vi "ICmainProgram.vi"() -> ()   [LabVIEW 2018]
uses:
  NetworkStream/NetworkStreamReceiverState.ctl
  NetworkStream/NetworkStreamData.ctl
  <vilib>/vision/Image Controls.llb/IMAQ Image.ctl
  NetworkStream/NetworkStreamStateMachineVariable.ctl
  <vilib>/dex/Stream Element Allocation Mode.ctl
  Shared program Control/MasterStatus.ctl
  StateMachine.ctl
  General Libraries/Photon Filtering.lvlib
  NetworkStream/NetworkStream.lvlib
  Tektronik3102/TektronikNetwork.lvlib
  Shared program Control/MySharedVariables.lvlib
panel:
  out "Network Stream State Indicator":T1
  out "output cluster":T2
  out "Session Hash":u64
  in  "Tab Control":enum32{"Camera", "Trigger", "configuration"}(tab)
  in  "exposure (us)":i32(slide) caption="exposure" scale=50.0..30000000.0
  in  "gain":i32(slide) scale=32.0..2047.0
  in  "sofware trigger":bool
  in  "live":bool
  in  "Save":bool
  in  "Trigger ON":bool
  out "Sequence Number":u64
  in  "Save Folder Path":path=path "D:/Data/Mai/test target"
  in  "VCD Properties":bool
  in  "Stop Button":bool
  out "error out":errorcluster
  in  "?":enum32{"IC control", "Data analysis", "graphs"}(tab)
  in  "ICImagingControl":refnum<k7>(container)
  out "Image":T3(plugin-control)
  in  "flush queue":bool
  in  "Flush Pile":bool
  in  "Mask ON":bool
  out "filtered \nFFT":dbl[][](graph)
  out "FFT":dbl[][](graph)
  in  "save image":bool
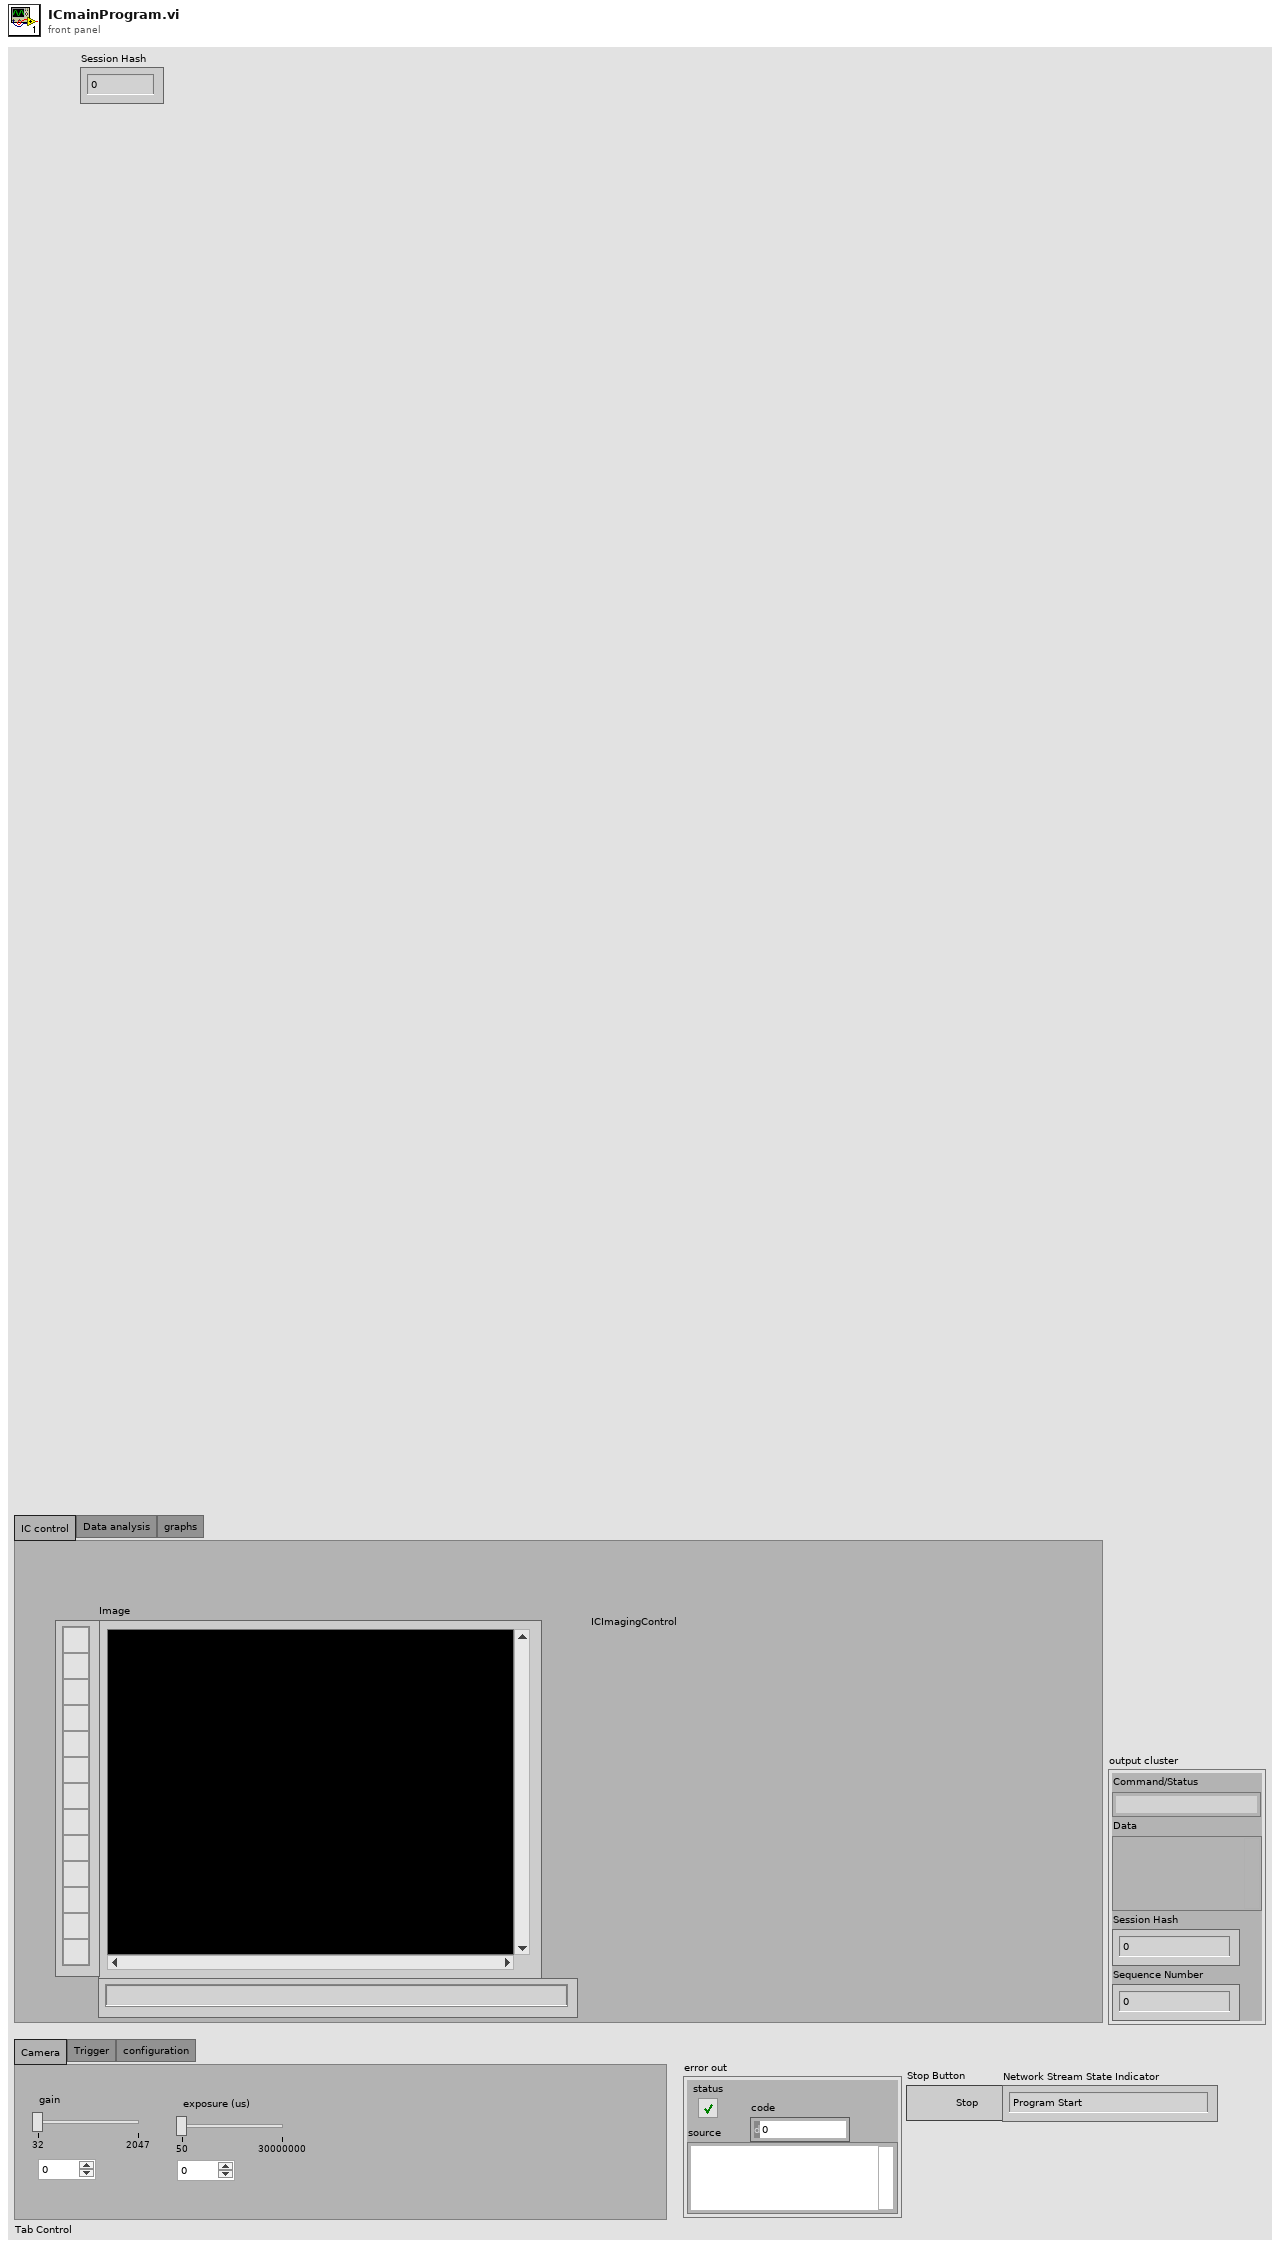
[diagram p1: front panel]
types:
  T1 = typedef "NetworkStream.lvlib/NetworkStreamReceiverState.ctl" = enum16{"Program Start", "Waiting for connection", "Connected", "Connection lost", "Exit", "Unhandled Exception"}
  T2 = typedef "NetworkStream.lvlib/NetworkStreamData.ctl" = cluster{"Command/Status":string, "Data":variant, "Session Hash":u64, "Sequence Number":u64}
  T3 = typedef "IMAQ Image.ctl" = refnum<image>
  T4 = typedef "NetworkStream.lvlib/NetworkStreamStateMachineVariable.ctl" = cluster{"Network Stream Reader Endpoint":refnum<k21>, "Last Received Sequence Number":u64}
  T5 = typedef "MySharedVariables.lvlib/MasterStatus.ctl" = cluster{"Camera done":bool, "Tektronik done":bool, "Motors done":bool, "Gage done":bool}[]
  T6 = cluster{"Image Out":T3, "Start time":dbl, "Stop time":dbl, "Index":i32}
  T7 = typedef "Stream Element Allocation Mode.ctl" = u32
  T8 = enum16{"Brightness", "Color Enable", "Contrast", "Exposure", "Focus", "Gain", "Gamma", "Hue", "Iris", "Pan", "Roll", "Saturation", "Sharpness", "Tilt", "Whitebalance", "Zoom", "Whitebalance Blue", "Whitebalance Red"}
  T9 = cluster{"Rows Per Strip":i32, "Photometric":i32, "Compression Type":i32}
  T10 = typedef "StateMachine.ctl" = enum16{"free running", "sequence recording", "run statistics"}
  T11 = cluster{"Image Out":T3, "SampleStartTime":dbl, "SampleEndTime":dbl, "Sequence Number":u64}
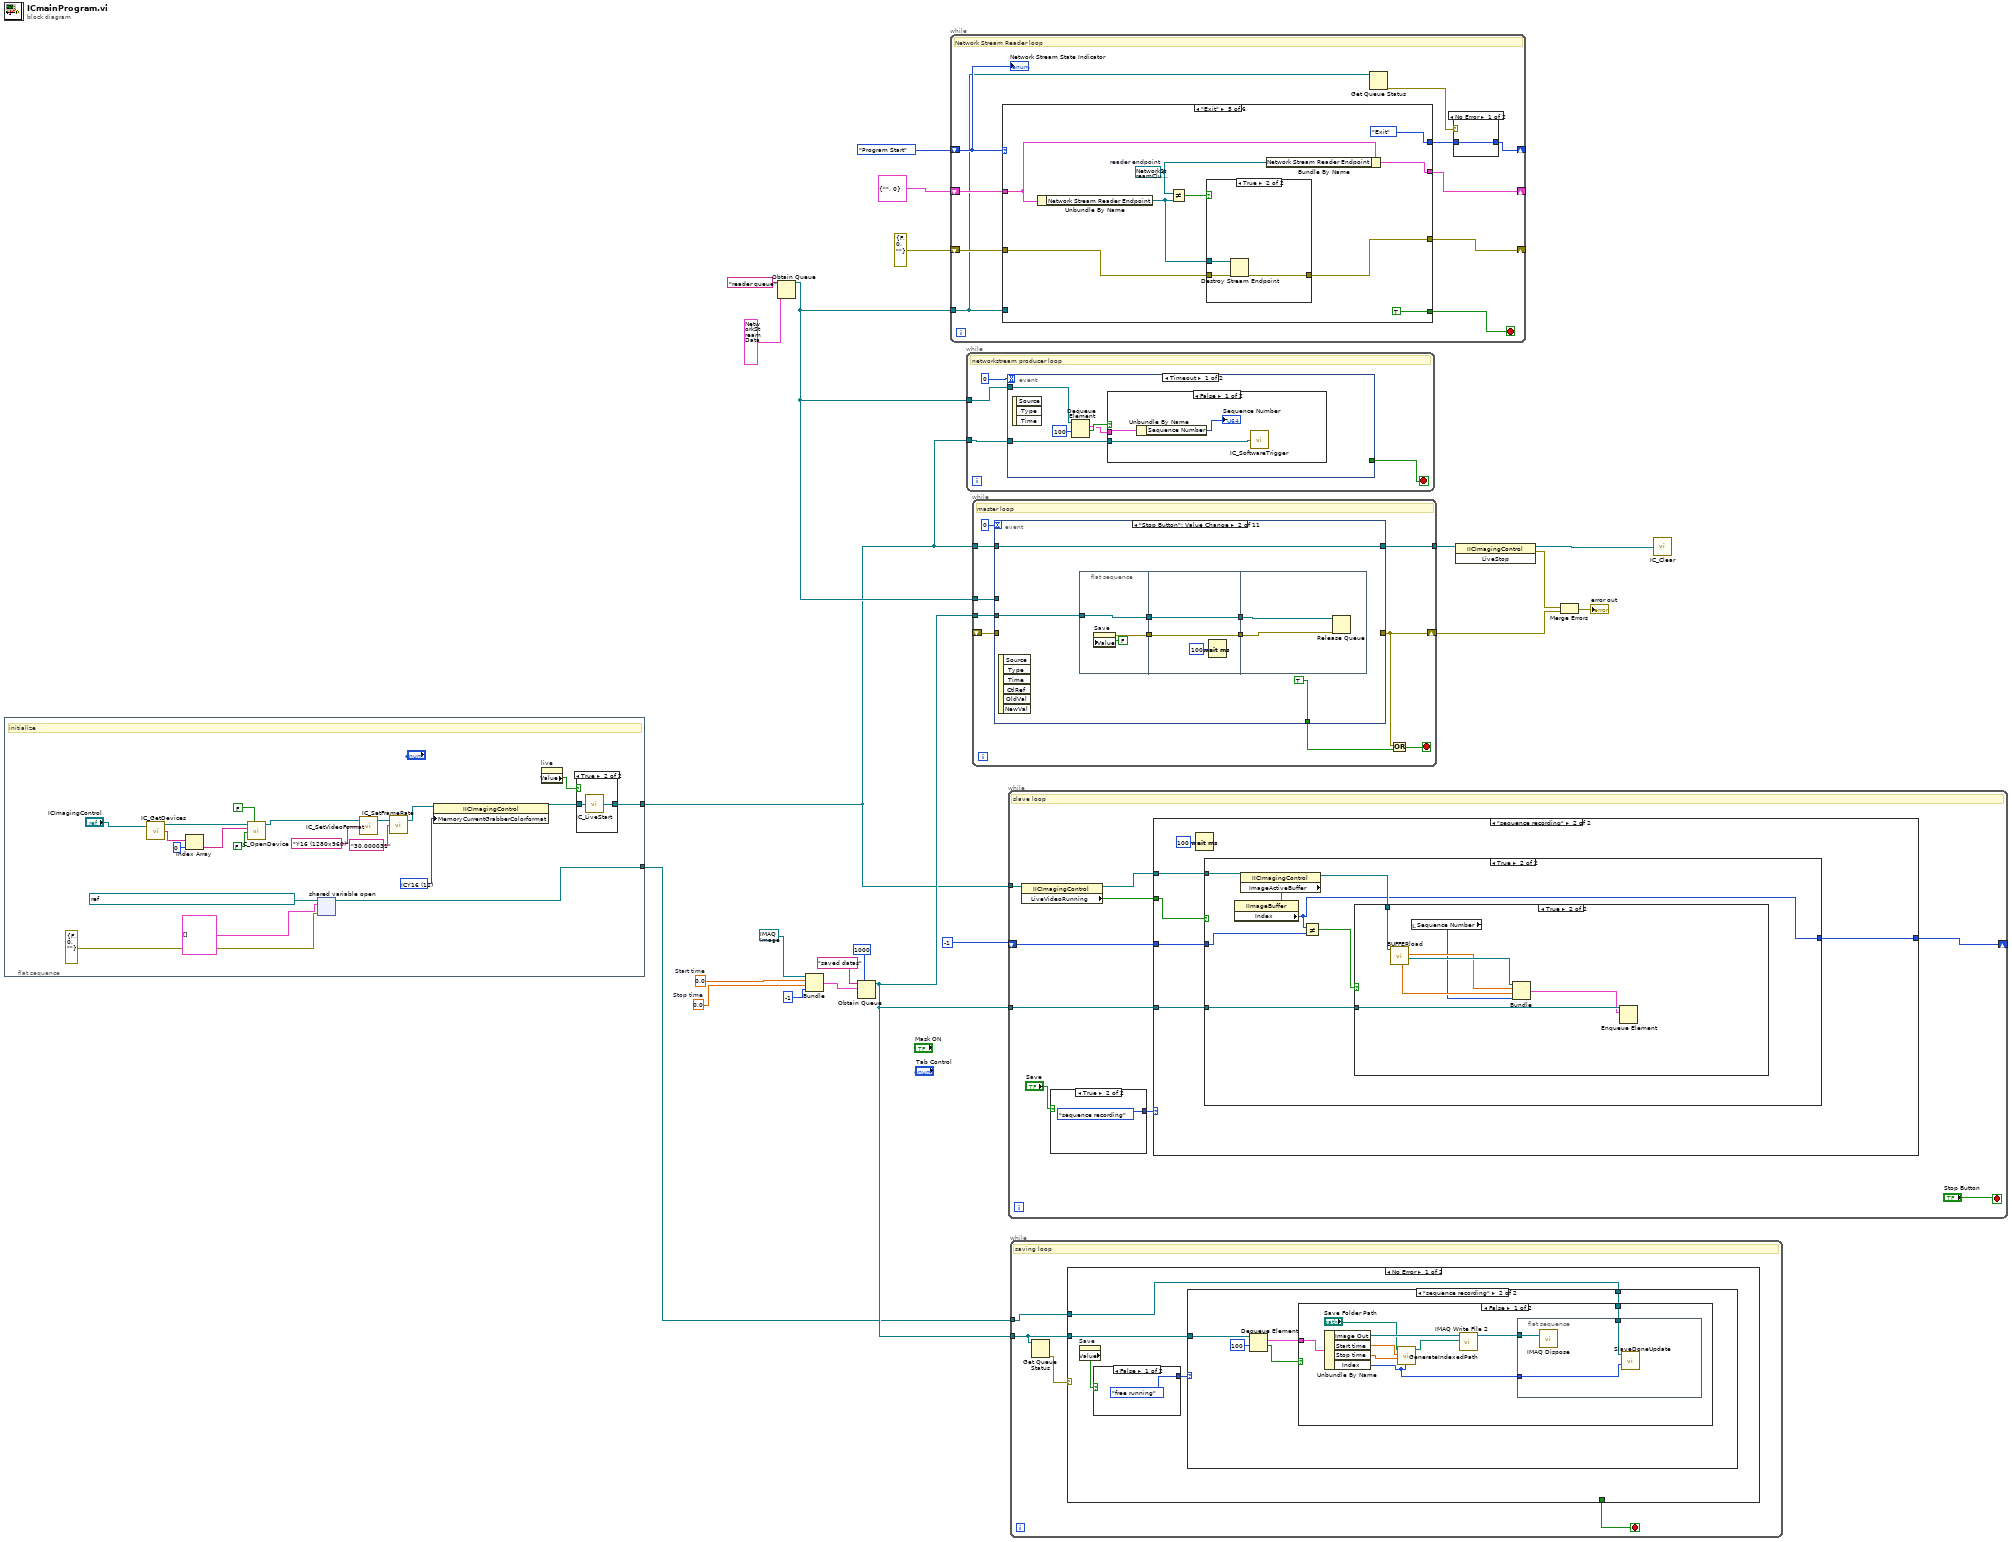
[diagram p0: block diagram]
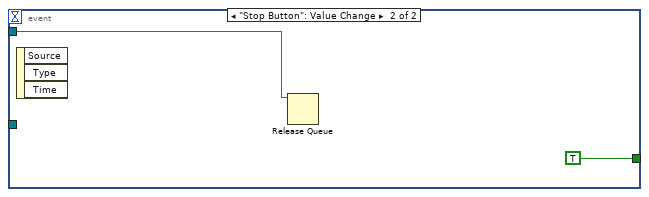
[diagram p3: hidden frame]
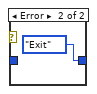
[diagram p4: hidden frame]
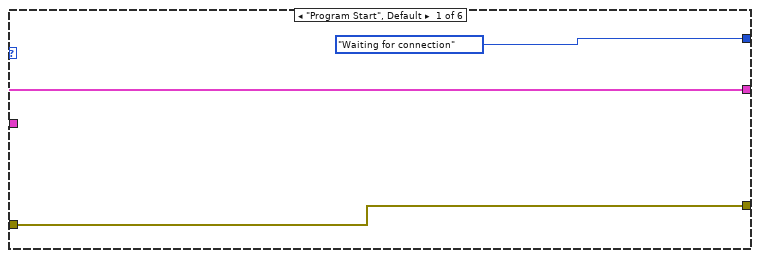
[diagram p5: hidden frame]
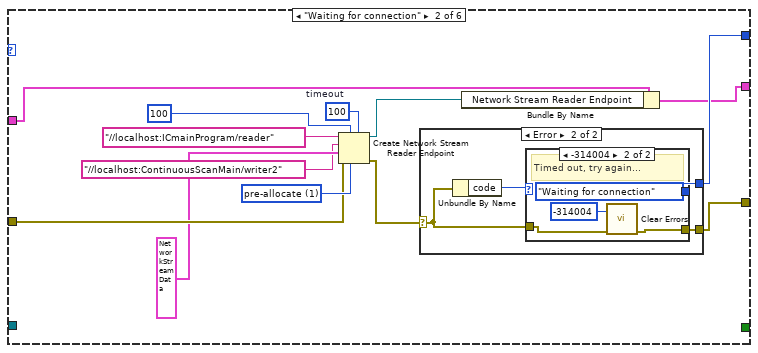
[diagram p6: hidden frame]
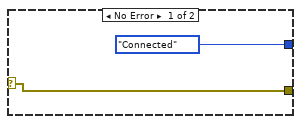
[diagram p7: hidden frame]
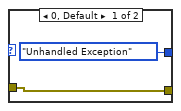
[diagram p8: hidden frame]
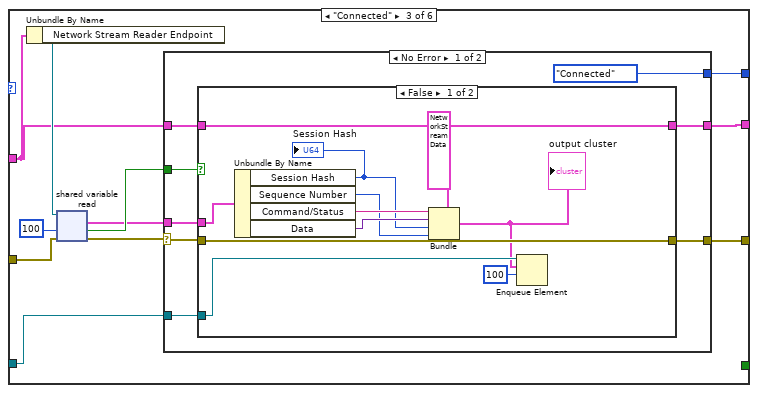
[diagram p9: hidden frame]
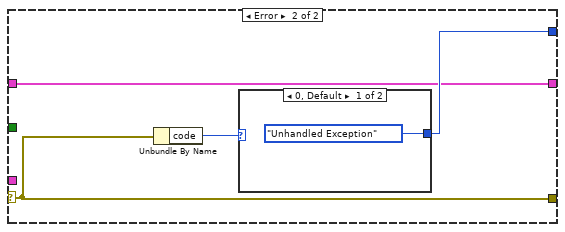
[diagram p11: hidden frame]
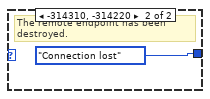
[diagram p12: hidden frame]
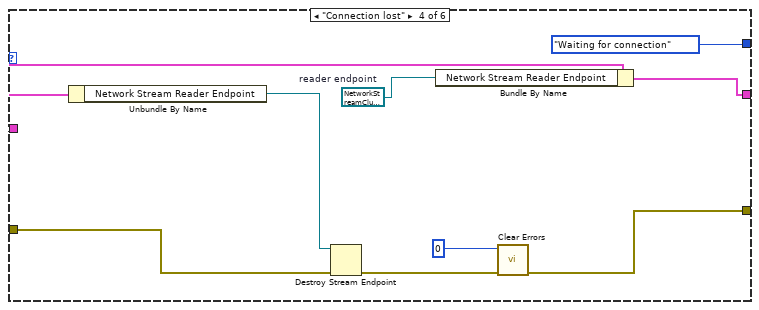
[diagram p13: hidden frame]
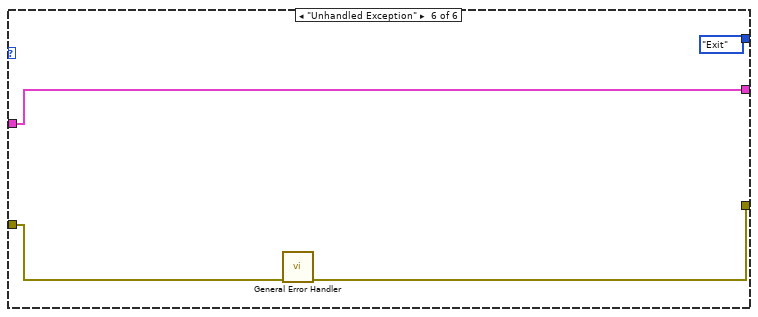
[diagram p15: hidden frame]
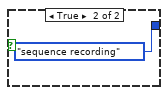
[diagram p16: hidden frame]
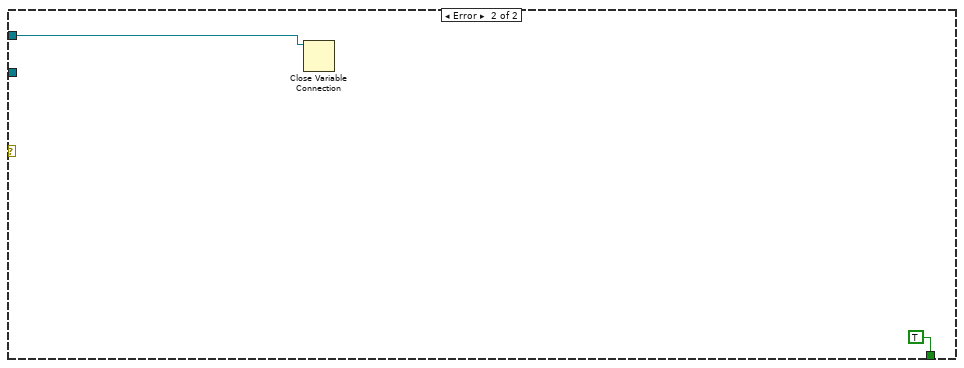
[diagram p19: hidden frame]
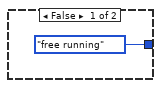
[diagram p20: hidden frame]
diagram:
  w10 = 0.0  # Stop time
  w14 = 0.0  # Start time
  n1 = flat-sequence {
    tunnel: [w28] -> w2
    tunnel: [w24] -> w1
    frame #0 {
      w32 = 11 items=["ICRGB32"=1, "ICRGB24"=2, "ICRGB565"=3, "ICRGB555"=4, "ICY8"=5, "ICUYVY"=6, "ICY800"=7, "ICYGB1"=8, "ICYGB0"=9, "ICBY8"=10, "ICY16"=11] ("MemoryCurrentGrabberColorformat")
      # "initialize"
      n2 = call <userlib>:"IC_GetDevices.vi"("ICImagingControl In"="ICImagingControl") -> ("ICImagingControl Out"=w39:refnum<k7>, "Devices"=w41:string[])  [unwired: 1 in, 1 out]
      n3 = Index Array(array=w41, index=0) -> (element=w38:string)
      n4 = call <userlib>:"IC_OpenDevice.vi"("Color"=FALSE, "Live"=FALSE, "Device"=w38, "ICImagingControl In"=w39) -> ("ICImagingControl Out"=w35:refnum<k7>)  [unwired: 2 in, 5 out]
      n5 = shared-variable-open(refnum<k21> "ni.var.psp://localhost/MySharedVariables/MasterStatusShared" ("shared variable refnum in"), errorcluster {"status"=FALSE, "code"=0, "source"=""} ("error in (no error)"), T5 [] ("MasterStatusShared")) -> (w24:refnum<k21>)  [unwired: 1 in, 1 out]
      n6 = call <userlib>:"IC_SetVideoFormat.vi"("VideoFormat"="Y16 (1280x960)", "ICImagingControl In"=w35) -> ("ICImagingControl Out"=w34:refnum<k7>)  [unwired: 1 in, 2 out]
      n7 = call <userlib>:"IC_SetFrameRate.vi"("FrameRate"="30,000031", "ICImagingControl In"=w34) -> ("ICImagingControl Out"=w33:refnum<k7>)  [unwired: 1 in, 1 out]
      n8 = property class="IICImagingControl"(reference=w33, "MemoryCurrentGrabberColorformat"=w32) -> (reference out=w29:refnum<k7>)  [unwired: 1 in, 1 out]
      n9 = property on="live" class="Bool (strict)"() -> ("Value"=w27:bool)  [unwired: 2 in, 2 out]
      n10 = case shown="True" w27 {
        tunnel: w29 -> [w43 w45]
        tunnel: [w43 w44] -> w28
        frame False {
        }
        frame True {
          n11 = call <userlib>:"IC_LiveStart.vi"("ICImagingControl 3"=w45) -> ("ICImagingControl 2"=w44:refnum<k7>)
        }
      }
    }
  }
  n12 = Obtain Queue(name (unnamed)="reader queue", element data type=T2 {"Command/Status"="", "Data"=variant, "Session Hash"=0, "Sequence Number"=0} ("NetworkStreamCluster")) -> (queue out=w3:refnum<queue>)  [unwired: 3 in, 2 out]
  n13 = Bundle("Image Out"=T3 refnum, "Start time"=w14, "Stop time"=w10, "Index"=-1) -> (w15:T6)  [unwired: 1 in]
  n14 = Obtain Queue(max queue size (-1, unlimited)=1000, name (unnamed)="saved datas", element data type=w15) -> (queue out=w13:refnum<queue>)  [unwired: 2 in, 2 out]
  n15 = while {
    shift-right: [w53] -> _
    shift-left: T4 {"Network Stream Reader Endpoint"="", "Last Received Sequence Number"=0} ("StateMachineVariable") -> [w55]
    shift-right: [w48] -> _
    shift-left: NetworkStreamReceiverState."Program Start" -> [w54]
    shift-right: [w52] -> _
    shift-left: errorcluster {"status"=FALSE, "code"=0, "source"=""} ("error in (no error)") -> [w50]
    tunnel: w3 -> [w46]
    stop <- w51 stop-if-true
    # "Network Stream Reader loop"
    n16 = case shown="\"Exit\"" w54 {
      tunnel: [NetworkStreamReceiverState."Waiting for connection" w69 w91 NetworkStreamReceiverState."Waiting for connection" NetworkStreamReceiverState."Exit" NetworkStreamReceiverState."Exit"] -> w49
      tunnel: [w59 w68 w92 w128 w141 w149] -> w52
      tunnel: [w58 w67 w89 w124 w134 w146] -> w53
      tunnel: [_ _ _ _ TRUE _] -> w51
      tunnel: w55 -> [w58 w65 w88 w125 w135 w146]
      tunnel: w50 -> [w59 w64 w87 w127 w136 w147]
      tunnel: w46 -> [_ _ w86 _ _ _]
      frame "Program Start", Default {
      }
      frame "Waiting for connection" {
        w66 = T7 1 items=["allocate as needed", "pre-allocate"] ("element allocation mode")
        w73 = 100  # timeout
        n17 = Create Network Stream Reader Endpoint(5:w73, 6:w66, 7:100 ("reader buffer size"), 8:w64, 9:T2 {"Command/Status"="", "Data"=variant, "Session Hash"=0, "Sequence Number"=0} ("NetworkStreamCluster"), 10:"//localhost:ContinuousScanMain/writer2" ("writer url"), 11:"//localhost:ICmainProgram/reader" ("reader name")) -> (0:w70:errorcluster, 3:w62:refnum<k21>)
        n18 = case shown="Error" w70 {
          selector: w70 -> [w74 w77]
          tunnel: [NetworkStreamReceiverState."Connected" w79] -> w69
          tunnel: [w74 w76] -> w68
          frame No Error {
          }
          frame Error {
            n19 = Unbundle By Name(w77) -> ("code"=w78:i32)
            n20 = case shown="-314004" w78 {
              tunnel: [NetworkStreamReceiverState."Unhandled Exception" NetworkStreamReceiverState."Waiting for connection"] -> w79
              tunnel: w77 -> [w80 w83]
              tunnel: [w80 w82] -> w76
              frame 0, Default {
              }
              frame -314004 {
                # "Timed out, try again..."
                n21 = call <vilib>:"Clear Errors.vi"("error in (no error)"=w83, "specific error code to clear (0: all)"=-314004) -> ("error out"=w82:errorcluster)  [unwired: 4 in, 1 out]
              }
            }
          }
        }
        n22 = Bundle By Name(cluster=w65, "Network Stream Reader Endpoint"=w62) -> (w67:T4)
      }
      frame "Connected" {
        n23 = Unbundle By Name(w88) -> ("Network Stream Reader Endpoint"=w90:refnum<k21>)
        n24 = shared-variable-read(w90, w87, 100 ("timeout ms (-1)")) -> (w93:errorcluster, w95:bool, w94:T2)  [unwired: 1 out]
        n25 = case shown="No Error" w93 {
          selector: w93 -> [w102 w121]
          tunnel: w95 -> [w104 _]
          tunnel: w94 -> [w103 _]
          tunnel: [w101 w121] -> w92
          tunnel: [NetworkStreamReceiverState."Connected" w119] -> w91
          tunnel: [w99 w118] -> w89
          tunnel: w88 -> [w98 w118]
          tunnel: w86 -> [w97 _]
          frame No Error {
            n26 = case shown="False" w104 {
              tunnel: [w111 w117] -> w101
              tunnel: w102 -> [w111 w117]
              tunnel: w103 -> [w115 _]
              tunnel: [w112 w116] -> w99
              tunnel: w98 -> [w112 w116]
              tunnel: w97 -> [w110 _]
              frame False {
                n27 = Unbundle By Name(w115) -> ("Session Hash"=w107:u64, "Sequence Number"=w106:u64, "Command/Status"=w114:string, "Data"=w113:variant)
                "Session Hash" <- w107
                n28 = Bundle(cluster=T2 {"Command/Status"="", "Data"=variant, "Session Hash"=0, "Sequence Number"=0} ("NetworkStreamCluster"), "Command/Status"=w114, "Data"=w113, "Session Hash"=w107, "Sequence Number"=w106) -> (w109:T2)
                "output cluster" <- w109
                n29 = Enqueue Element(queue=w110, element=w109, timeout in ms (-1)=100) -> ()  [unwired: 1 in, 3 out]
              }
              frame True {
              }
            }
          }
          frame Error {
            n30 = Unbundle By Name(w121) -> ("code"=w120:i32)
            n31 = case shown="0, Default" w120 {
              tunnel: [NetworkStreamReceiverState."Unhandled Exception" NetworkStreamReceiverState."Connection lost"] -> w119
              frame 0, Default {
              }
              frame -314310, -314220 {
                # "The remote endpoint has been destroyed."
              }
            }
          }
        }
      }
      frame "Connection lost" {
        w131 = refnum<k21> refnum  # reader endpoint
        n32 = Unbundle By Name(w125) -> ("Network Stream Reader Endpoint"=w126:refnum<k21>)
        n33 = Destroy Stream Endpoint(8:w127, 11:w126) -> (0:w130:errorcluster)
        n34 = Bundle By Name(cluster=w125, "Network Stream Reader Endpoint"=w131) -> (w124:T4)
        n35 = call <vilib>:"Clear Errors.vi"("error in (no error)"=w130, "specific error code to clear (0: all)"=0) -> ("error out"=w128:errorcluster)  [unwired: 4 in, 1 out]
      }
      frame "Exit" {
        w137 = refnum<k21> refnum  # reader endpoint
        n36 = Unbundle By Name(w135) -> ("Network Stream Reader Endpoint"=w133:refnum<k21>)
        n37 = Not Equal?(x=w137, y=w133) -> (x != y?=w139:bool)
        n38 = case shown="True" w139 {
          tunnel: [w142 w145] -> w141
          tunnel: w136 -> [w142 w144]
          tunnel: w133 -> [_ w143]
          frame False {
          }
          frame True {
            n39 = Destroy Stream Endpoint(8:w144, 11:w143) -> (0:w145:errorcluster)
          }
        }
        n40 = Bundle By Name(cluster=w135, "Network Stream Reader Endpoint"=w137) -> (w134:T4)
      }
      frame "Unhandled Exception" {
        n41 = call <vilib>:"General Error Handler.vi"("error in (no error)"=w147) -> ("error out"=w149:errorcluster)  [unwired: 10 in, 4 out]
      }
    }
    n42 = Get Queue Status(queue=w46) -> (error out=w47:errorcluster)  [unwired: 2 in, 7 out]
    n43 = case shown="No Error" w47 {
      tunnel: w49 -> [w56 _]
      tunnel: [w56 NetworkStreamReceiverState."Exit"] -> w48
      frame No Error {
      }
      frame Error {
      }
    }
    "Network Stream State Indicator" <- w54
  }
  n44 = while {
    tunnel: w3 -> [w152]
    tunnel: w2 -> [w150]
    stop <- w151 stop-if-true
    # "networkstream producer loop"
    n45 = event shown="[0] Timeout" {
      selector: _ -> [_ _]
      dyn-events: _ -> [_ _]
      timeout: 0 -> [_ _]
      tunnel: w152 -> [w155 w163]
      tunnel: [_ TRUE] -> w151
      tunnel: w150 -> [w154 _]
      event Timeout {
        n46 = event-data() -> ()  [unwired: 1 in, 3 out]
        n47 = Dequeue Element(queue=w155, timeout in ms (-1)=100) -> (element=w156:T2, timed out?=w157:bool)  [unwired: 1 in, 2 out]
        n48 = case shown="False" w157 {
          tunnel: w156 -> [w161 _]
          tunnel: w154 -> [w159 _]
          frame False {
            n49 = Unbundle By Name(w161) -> ("Sequence Number"=→"Sequence Number":u64)
            n50 = call <userlib>:"IC_SoftwareTrigger.vi"("ICImagingControl 3"=w159) -> ()  [unwired: 1 out]
          }
          frame True {
          }
        }
      }
      event "Stop Button": Value Change {
        n51 = event-data() -> ()  [unwired: 1 in, 3 out]
        n52 = Release Queue(queue=w163) -> ()  [unwired: 2 in, 3 out]
      }
    }
  }
  n53 = while {
    tunnel: w2 -> [w171]
    tunnel: [w172] -> w22
    shift-right: [w169] -> w19
    shift-left: _ -> [w170]
    tunnel: w13 -> [w166]
    tunnel: w3 -> [w165]
    stop <- w168 stop-if-true
    # "master loop"
    n54 = event shown="[1] \"Stop Button\": Value Change" {
      selector: _ -> [_ _ _ _ _ _ _ _ _ _ _]
      dyn-events: _ -> [_ _ _ _ _ _ _ _ _ _ _]
      timeout: 0 -> [_ _ _ _ _ _ _ _ _ _ _]
      tunnel: [_ TRUE _ _ _ _ _ _ _ _ _] -> w167
      tunnel: [w173 w180 _ w192 w194 w206 w209 _ w218 _ w235] -> w172
      tunnel: w171 -> [w173 w180 _ w193 w195 w207 w208 _ w219 w229 w236]
      tunnel: [w174 _ _ _ w196 w204 w210 _ w217 w232 w234] -> w169
      tunnel: w170 -> [w174 _ w190 _ w196 w205 w211 _ w216 w222 w234]
      tunnel: w166 -> [_ w175 w191 _ _ _ _ w214 _ _ _]
      tunnel: w165 -> [_ _ _ _ _ _ _ _ _ _ _]
      event Timeout {
        n55 = event-data() -> ()  [unwired: 1 in, 3 out]
      }
      event "Stop Button": Value Change {
        n56 = event-data() -> ()  [unwired: 1 in, 6 out]
        n57 = flat-sequence {
          tunnel: [w183] -> w179
          tunnel: [w182] -> w176
          tunnel: w175 -> [w182]
          tunnel: w179 -> [w187]
          tunnel: [w187] -> w178
          tunnel: [w186] -> w177
          tunnel: w176 -> [w186]
          tunnel: w178 -> [w188]
          tunnel: w177 -> [w189]
          frame #0 {
            n58 = property on="Save" class="Bool (strict)"("Value"=FALSE ("Save")) -> (error out=w183:errorcluster)  [unwired: 2 in, 1 out]
          }
          frame #1 {
            n59 = Wait (ms)(milliseconds to wait=u32 100) -> ()  [unwired: 1 out]
          }
          frame #2 {
            n60 = Release Queue(queue=w189, error in (no error)=w188) -> ()  [unwired: 1 in, 3 out]
          }
        }
      }
      event "flush queue": Value Change {
        n61 = event-data() -> ()  [unwired: 1 in, 6 out]
        n62 = Flush Queue(queue=w191, error in (no error)=w190) -> ()  [unwired: 3 out]
      }
      event "VCD Properties": Value Change {
        n63 = event-data() -> ()  [unwired: 1 in, 6 out]
        n64 = invoke class="IICImagingControl" method="ShowPropertyDialog"(reference=w193) -> (reference out=w192:refnum<k7>)  [unwired: 2 in, 2 out]
      }
      event "live": Value Change {
        n65 = event-data() -> ("NewVal"=w197:bool)  [unwired: 1 in, 5 out]
        n66 = case shown="True" w197 {
          tunnel: w195 -> [w199 w201]
          tunnel: [w198 w200] -> w194
          frame False {
            n67 = invoke class="IICImagingControl" method="LiveStop"(reference=w199) -> (reference out=w198:refnum<k7>)  [unwired: 2 in, 2 out]
          }
          frame True {
            n68 = call <userlib>:"IC_LiveStart.vi"("ICImagingControl 3"=w201) -> ("ICImagingControl 2"=w200:refnum<k7>)
          }
        }
      }
      event "exposure (us)": Value Change {
        n69 = event-data() -> ()  [unwired: 1 in, 6 out]
        n70 = call <userlib>:"IC_SetPropertyValue.vi"("Error In (no error)"=w205, "Value"="exposure (us)", "Property"=T8."Exposure", "ICImagingControl In"=w207) -> ("Error Out"=w204:errorcluster, "ICImagingControl Out"=w206:refnum<k7>)
      }
      event "gain": Value Change {
        n71 = event-data() -> ()  [unwired: 1 in, 6 out]
        n72 = call <userlib>:"IC_SetPropertyValue.vi"("Error In (no error)"=w211, "Value"="gain", "Property"=T8."Gain", "ICImagingControl In"=w208) -> ("Error Out"=w210:errorcluster, "ICImagingControl Out"=w209:refnum<k7>)
      }
      event "Flush Pile": Value Change {
        n73 = event-data() -> ()  [unwired: 1 in, 6 out]
        n74 = Flush Queue(queue=w214) -> ()  [unwired: 1 in, 3 out]
      }
      event "Trigger ON": Value Change {
        n75 = event-data() -> ("NewVal"=w215:bool)  [unwired: 1 in, 5 out]
        n76 = call <userlib>:"IC_SetExtenalTrigger.vi"("Error In (no error)"=w216, "Trigger"=w215, "ICImagingControl In"=w219) -> ("Error Out"=w217:errorcluster, "ICImagingControl Out"=w218:refnum<k7>)
      }
      event "save image": Value Change {
        n77 = event-data() -> ()  [unwired: 1 in, 6 out]
        n78 = invoke class="IICImagingControl" method="LiveStop"(reference=w229) -> (reference out=w228:refnum<k7>)  [unwired: 2 in, 2 out]
        n79 = property on="Save Folder Path" class="Path"() -> ("Value"=w225:path)  [unwired: 2 in, 2 out]
        n80 = property class="IICImagingControl" props=["ImageActiveBuffer"](reference=w228) -> (reference out=w227:refnum<k7>)  [unwired: 1 in, 2 out]
        n81 = File Dialog(4:".tiff" ("pattern label"), 7:"select file name" ("prompt"), 8:w222, 11:w225) -> (0:w221:errorcluster, 3:w224:path)  [unwired: 1 in, 4 out]
        n82 = call <userlib>:"IC_ActiveBuffer_to_IMAQ.vi"("ICImagingControl In"=w227) -> ("Image Out"=w226:T3)  [unwired: 2 in, 3 out]
        n83 = call-poly "IMAQ Write File 2"("error in (no error)"=w221, "TIFF Options"=T9 {"Rows Per Strip"=0, "Photometric"=1, "Compression Type"=0}, "File Path"=w224, "Image"=w226) -> ("error out"=w233:errorcluster, "Image Out (duplicate)"=w231:T3)  [unwired: 6 in]
        n84 = call "IMAQ Dispose"("Image"=w231, "error in (no error)"=w233) -> ("error out"=w232:errorcluster)  [unwired: 4 in]
      }
      event "sofware trigger": Value Change {
        n85 = event-data() -> ()  [unwired: 1 in, 6 out]
        n86 = call <userlib>:"IC_SoftwareTrigger.vi"("ICImagingControl 3"=w236) -> ("ICImagingControl 2"=w235:refnum<k7>)
      }
    }
    n87 = Or(x=w169, y=w167) -> (x .or. y?=w168:bool)
  }
  n88 = while {
    tunnel: w2 -> [w240]
    shift-right: [w243] -> _
    shift-left: -1 ("Index") -> [w245]
    tunnel: w13 -> [w237]
    stop <- "Stop Button" stop-if-true
    # "slave loop"
    n89 = property class="IICImagingControl"(reference=w240) -> (reference out=w238:refnum<k7>, "LiveVideoRunning"=w239:bool)  [unwired: 1 in, 1 out]
    n90 = case shown="True" "Save" {
      tunnel: [StateMachine."free running" ("loop state") StateMachine."sequence recording" ("loop state")] -> w241
      frame False {
      }
      frame True {
      }
    }
    n91 = case shown="\"sequence recording\"" w241 {
      tunnel: w245 -> [w251 w276]
      tunnel: [w250 w274] -> w243
      tunnel: w239 -> [w249 w275]
      tunnel: w238 -> [w248 w277]
      tunnel: w237 -> [_ w273]
      frame "free running", Default {
        n92 = case shown="True" w249 {
          tunnel: w251 -> [w252 w258]
          tunnel: [w252 w255] -> w250
          tunnel: w248 -> [_ w254]
          frame False {
          }
          frame True {
            n93 = property class="IICImagingControl"(reference=w254) -> (reference out=w256:refnum<k7>, "ImageActiveBuffer"=w257:refnum<k7>)  [unwired: 1 in, 1 out]
            n94 = property class="IImageBuffer"(reference=w257) -> ("Index"=w255:i32)  [unwired: 1 in, 2 out]
            n95 = Not Equal?(x=w255, y=w258) -> (x != y?=w253:bool)
            n96 = case shown="True" w253 {
              tunnel: w256 -> [_ w263]
              frame False {
                n97 = Wait (ms)(milliseconds to wait=u32 200) -> ()  [unwired: 1 out]
              }
              frame True {
                n98 = call "BUFFERload.vi"("ICImagingControl In"=w263) -> ("Image Out"=w260:T3, "SampleStartTime"=w262:dbl)  [unwired: 6 in, 3 out]
                n99 = flat-sequence {
                  tunnel: w260 -> [w270]
                  tunnel: [w270] -> w261
                  tunnel: w262 -> [_]
                  tunnel: w261 -> [w271]
                  frame #0 {
                    n100 = call "IMAQ ImageToArray"("Image"=w270) -> ("Image Pixels (U16)"=w269:u16[][])  [unwired: 3 in, 4 out]
                    n101 = control-ref of="FFT"() -> (w266:refnum<vi>)
                    n102 = Transpose 2D Array(2D array=w269) -> (transposed array=w268:u16[][])
                    n103 = To Double Precision Float(number=w268) -> (double precision float=w267:dbl[][])
                    n104 = call "GetTaggedPhotons.vi"("FFT reference"=w266, "double precision float"=w267) -> ("FFT modulous"=→"FFT":dbl[][], "tagged photons"=→"filtered \nFFT":dbl[][])  [unwired: 6 in, 2 out]
                    "Image" <- w270
                  }
                  frame #1 {
                    n105 = call "IMAQ Dispose"("Image"=w271) -> ()  [unwired: 5 in, 1 out]
                  }
                }
              }
            }
          }
        }
      }
      frame "sequence recording" {
        n106 = Wait (ms)(milliseconds to wait=u32 100) -> ()  [unwired: 1 out]
        n107 = case shown="True" w275 {
          tunnel: [w278 w281] -> w274
          tunnel: w277 -> [_ w285]
          tunnel: w276 -> [w278 w280]
          tunnel: w273 -> [_ w283]
          frame False {
          }
          frame True {
            n108 = property class="IICImagingControl"(reference=w285) -> (reference out=w282:refnum<k7>, "ImageActiveBuffer"=w284:refnum<k7>)  [unwired: 1 in, 1 out]
            n109 = property class="IImageBuffer"(reference=w284) -> ("Index"=w281:i32)  [unwired: 1 in, 2 out]
            n110 = Not Equal?(x=w281, y=w280) -> (x != y?=w279:bool)
            n111 = case shown="True" w279 {
              tunnel: w283 -> [_ w288]
              tunnel: w282 -> [_ w292]
              frame False {
              }
              frame True {
                n112 = call "BUFFERload.vi"("ICImagingControl In"=w292) -> ("Image Out"=w291:T3, "SampleStartTime"=w290:dbl, "SampleEndTime"=w289:dbl)  [unwired: 6 in, 2 out]
                n113 = local read "Sequence Number"() -> (w286:u64)
                n114 = Bundle("Image Out"=w291, "SampleStartTime"=w290, "SampleEndTime"=w289, "Sequence Number"=w286) -> (w287:T11)  [unwired: 1 in]
                n115 = Enqueue Element(queue=w288, element=w287) -> ()  [unwired: 2 in, 3 out]
              }
            }
          }
        }
      }
    }
  }
  n116 = while {
    tunnel: w13 -> [w296]
    tunnel: w1 -> [w293]
    stop <- w294 stop-if-true
    # "saving loop"
    n117 = Get Queue Status(queue=w296) -> (error out=w295:errorcluster)  [unwired: 2 in, 7 out]
    n118 = case shown="No Error" w295 {
      tunnel: w296 -> [w300 _]
      tunnel: [_ TRUE] -> w294
      tunnel: w293 -> [w297 w320]
      frame No Error {
        n119 = property on="Save" class="Bool (strict)"() -> ("Value"=w298:bool)  [unwired: 2 in, 2 out]
        n120 = case shown="False" w298 {
          tunnel: [StateMachine."free running" ("loop state") StateMachine."sequence recording" ("loop state")] -> w299
          frame False {
          }
          frame True {
          }
        }
        n121 = case shown="\"sequence recording\"" w299 {
          tunnel: w300 -> [_ w306]
          tunnel: w297 -> [_ w303]
          frame "free running", Default {
          }
          frame "sequence recording" {
            n122 = Dequeue Element(queue=w306, timeout in ms (-1)=100) -> (element=w305:T6, timed out?=w304:bool)  [unwired: 1 in, 2 out]
            n123 = case shown="False" w304 {
              tunnel: w305 -> [w316 _]
              tunnel: w303 -> [w308 _]
              frame False {
                n124 = Unbundle By Name(w316) -> ("Image Out"=w315:T3, "Start time"=w312:dbl, "Stop time"=w313:dbl, "Index"=w309:i32)
                n125 = call "GenerateIndexedPath.vi"("number"=w309, "stop"=w313, "start"=w312, "input folder"="Save Folder Path") -> ("output path"=w311:path)  [unwired: 7 in]
                n126 = call-poly "IMAQ Write File 2"("File Path"=w311, "Image"=w315) -> ("Image Out (duplicate)"=w314:T3)  [unwired: 8 in, 1 out]
                n127 = flat-sequence {
                  tunnel: w314 -> [w319]
                  tunnel: w309 -> [w318]
                  tunnel: w308 -> [w317]
                  frame #0 {
                    n128 = call "IMAQ Dispose"("Image"=w319) -> ()  [unwired: 5 in, 1 out]
                    n129 = call "SlaveDoneUpdate.vi"("shared index"=w318, "shared variable"=w317) -> ()  [unwired: 10 in]
                  }
                }
              }
              frame True {
              }
            }
          }
        }
      }
      frame Error {
        n130 = Close Variable Connection(11:w320) -> ()  [unwired: 1 in, 1 out]
      }
    }
  }
  n131 = invoke class="IICImagingControl" method="LiveStop"(reference=w22) -> (reference out=w21:refnum<k7>, error out=w18:errorcluster)  [unwired: 2 in, 1 out]
  n132 = Merge Errors(w18, w19) -> (→"error out":errorcluster)
  n133 = call <userlib>:"IC_Clear.vi"("ICImagingControl 2"=w21) -> ()  [unwired: 1 out]
